vi "Selete_SW_Cmd.vi"(0 "VISA资源名称 2":refnum<visa-resource-name>, 1 "组合框":string(combo), 2 "H_32":bool[](array[boolean]), 3 "L_32":bool[](array[boolean]), 4 "64 SW OUT":bool[](array[boolean]), 5 "error in (no error)":errorcluster caption="错误输入（无错误）") -> (14 "VISA资源名称":refnum<visa-resource-name>, 19 "error out":errorcluster caption="错误输出")   [LabVIEW 2018]
panel:
  out "OpenStr":string
  out "ColseStr":string
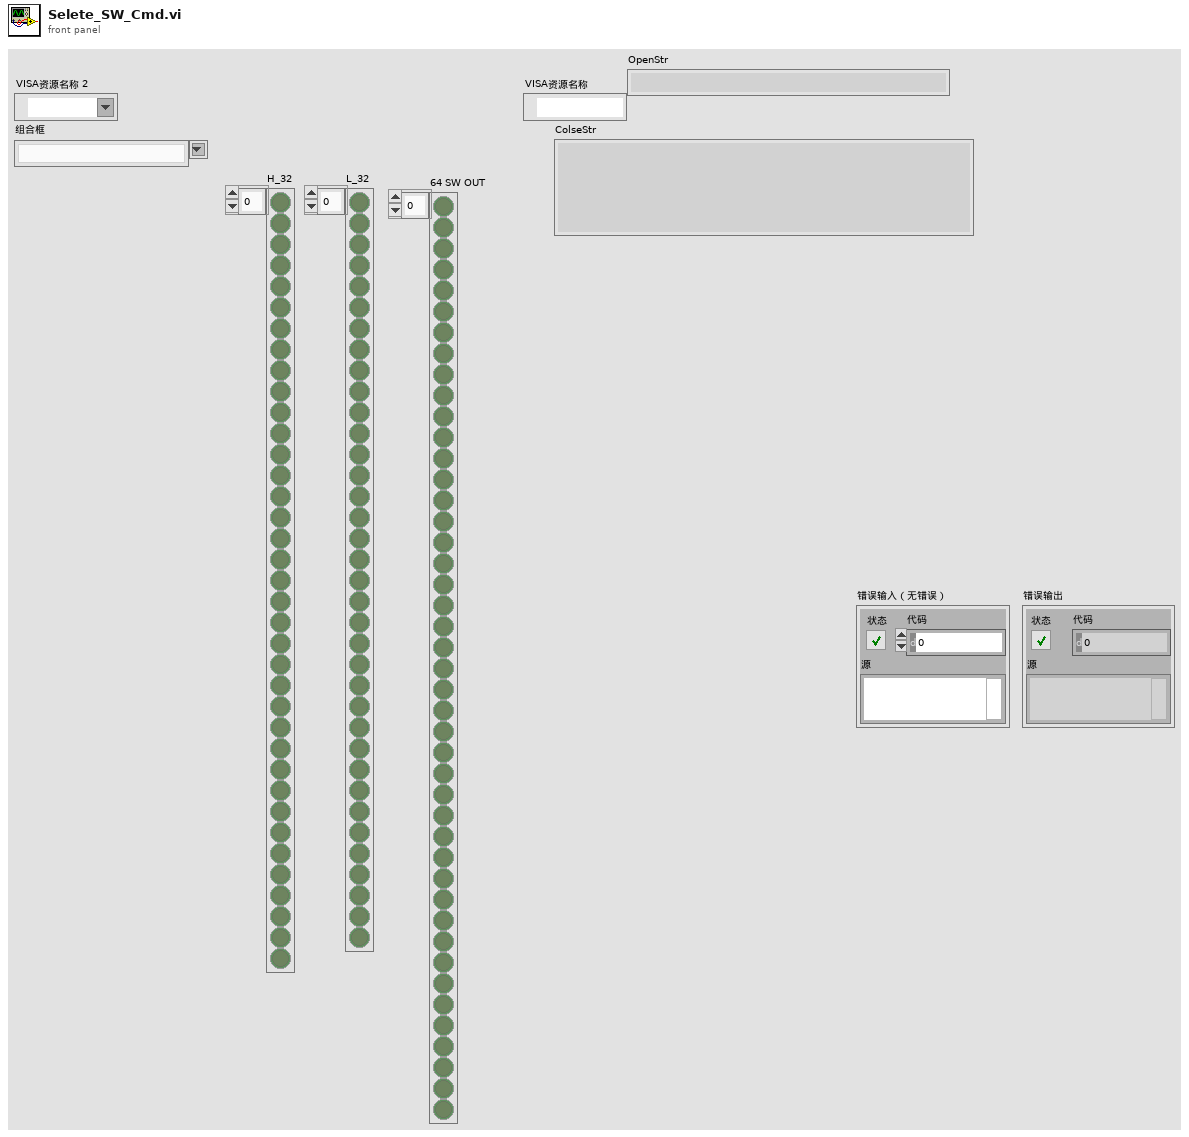
[diagram p1: front panel]
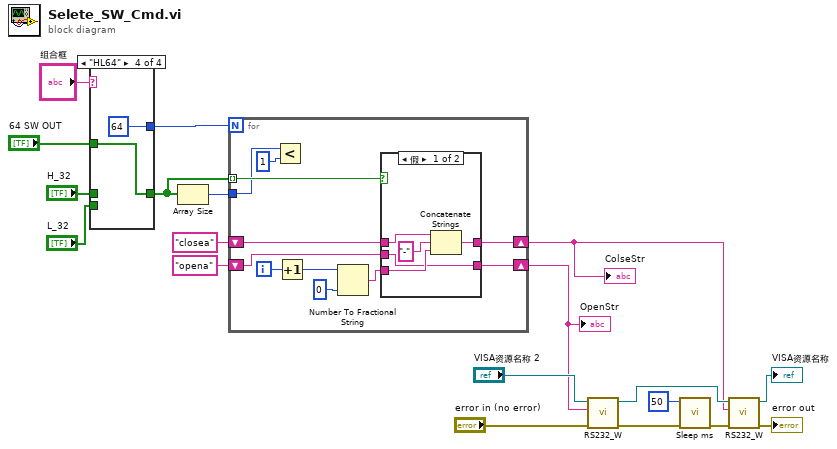
[diagram p0: block diagram]
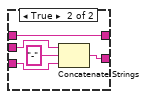
[diagram p2: hidden frame]
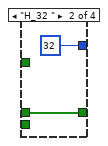
[diagram p4: hidden frame]
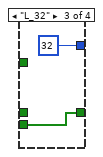
[diagram p5: hidden frame]
diagram:
  n1 = case shown="\"HL64\"" "组合框" {
    tunnel: "H_32" -> [_ w21 _ _]
    tunnel: "L_32" -> [_ _ w23 _]
    tunnel: "64 SW OUT" -> [_ _ _ w25]
    tunnel: [_ w21 w23 w25] -> w4
    tunnel: [_ 32 32 64] -> w15
    frame "假", Default {
    }
    frame "H_32 " {
    }
    frame "L_32" {
    }
    frame "HL64" {
    }
  }
  n2 = Array Size(array=w4) -> (size(s)=w3:i32)
  n3 = for {
    N: w15 -> [_]
    tunnel: w4 -> [w31] mode=indexing
    shift-right: [w32] -> w2
    shift-left: "opena" -> [w30]
    shift-right: [w27] -> w1
    shift-left: "closea" -> [w29]
    tunnel: w3 -> [w26]
    i -> [w36]
    n4 = Less?(x=w26, y=1) -> ()  [unwired: 1 out]
    n5 = Increment(x=w36) -> (x+1=w35:i32)
    n6 = Number To Fractional String(number=w35, precision (6)=i16 0 ("精度(6)")) -> (F-format string=w33:string)  [unwired: 2 in]
    n7 = case shown="假" w31 {
      tunnel: w33 -> [w40 w44]
      tunnel: [w38 w46] -> w32
      tunnel: w30 -> [w38 w42]
      tunnel: w29 -> [w37 w43]
      tunnel: [w39 w43] -> w27
      frame False {
        n8 = Concatenate Strings(w37, "-", w40) -> (w39:string)
      }
      frame True {
        n9 = Concatenate Strings(w42, "-", w44) -> (w46:string)
      }
    }
  }
  "ColseStr" <- w1
  "OpenStr" <- w2
  n10 = call "RS232_W.vi"("error in (no error)"="error in (no error)", "CMD"=w2, "VISA资源名称"="VISA资源名称 2") -> ("error out"=w9:errorcluster, "VISA资源名称输出"=w11:refnum<visa-resource-name>)  [unwired: 6 in, 1 out]
  n11 = call "Sleep ms.vi"("error in (no error)"=w9, "等待时间（毫秒）"=u32 50) -> ("error out"=w8:errorcluster)  [unwired: 9 in]
  n12 = call "RS232_W.vi"("error in (no error)"=w8, "CMD"=w1, "VISA资源名称"=w11) -> ("error out"=→"error out":errorcluster, "VISA资源名称输出"=→"VISA资源名称":refnum<visa-resource-name>)  [unwired: 6 in, 1 out]
